vi "Adjust Graph Cursor Index.vi"(5 "index adjustment":i32, 7 "Plot 0 samples":i64, 8 "error in":errorcluster, 11 "WaveformGraph in":refnum<vi>) -> (0 "error out":errorcluster, 2 "adjusted index":i32)   [LabVIEW 2018, in "NI_TDMS File Viewer.lvlib"]
uses:
  NI_TDMS File Viewer.lvlib
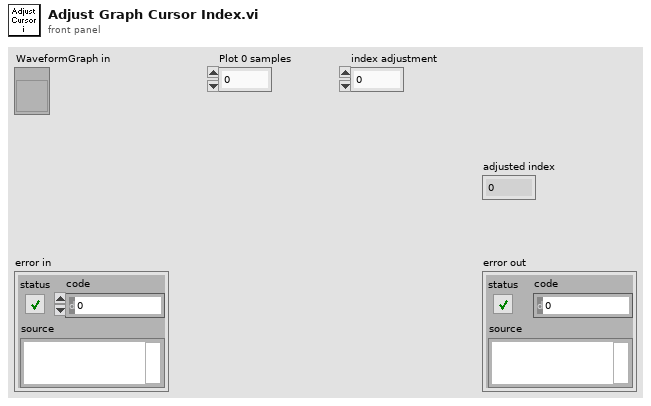
[diagram p1: front panel]
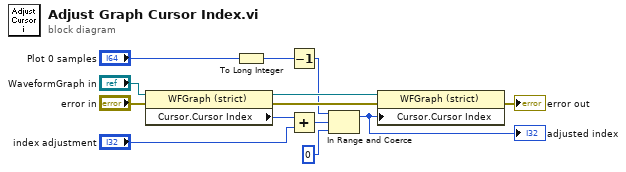
[diagram p0: block diagram]
diagram:
  n1 = property on="Property Node" class="WFGraph (strict)"(reference="WaveformGraph in", error in="error in") -> (reference out=w7:refnum<vi>, error out=w12:errorcluster, "Cursor.Cursor Index"=w9:i32)
  n2 = To Long Integer(number="Plot 0 samples") -> (32bit integer=w3:i32)
  n3 = Decrement(x=w3) -> (x-1=w1:i32)
  n4 = Add(x=w9, y="index adjustment") -> (x+y=w5:i32)
  n5 = In Range and Coerce(upper limit=w1, x=w5, lower limit=0 ("y")) -> (coerced(x)=w2:i32)  [unwired: 1 out]
  "adjusted index" <- w2
  n6 = property on="Property Node" class="WFGraph (strict)"(reference=w7, error in=w12, "Cursor.Cursor Index"=w2) -> (error out=→"error out":errorcluster)  [unwired: 1 out]
